vi "Find Connection.vi"(9 "Z":dbl, 10 "X":dbl, 11 "All Lines":T1) -> (0 "Distance to nearest":dbl, 1 "Index on Line":i32, 2 "Nearest Line":i32, 3 "Line found?":bool, 4 "Bool to number":u32, 5 "Z Coonnection":dbl, 7 "X Connection":dbl)   [LabVIEW 2014, in "Map Data.lvlib"]
uses:
  Map Data.lvlib
  All-Lines.ctl
  LineCluster.ctl
  LineConnection.ctl
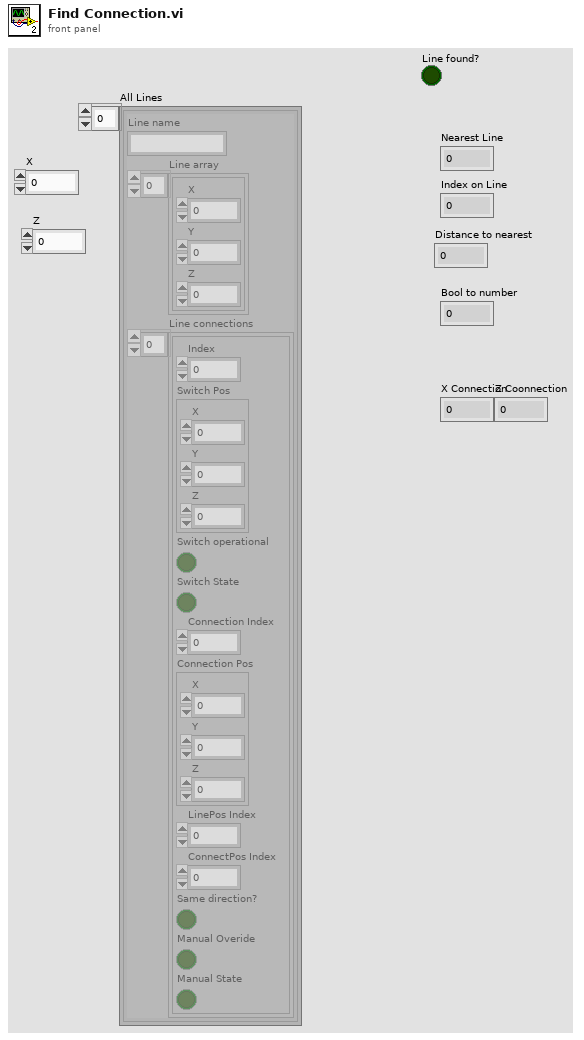
[diagram p1: front panel]
types:
  T1 = typedef "Map Data.lvlib/All-Lines.ctl" = T2[]
  T2 = typedef "Map Data.lvlib/LineCluster.ctl" = cluster{"Line name":string, "Line array":cluster{"X":dbl, "Y":dbl, "Z":dbl}[], "Line connections":T3[]}
  T3 = typedef "Map Data.lvlib/LineConnection.ctl" = cluster{"Index":i32, "Switch Pos":cluster{"X":dbl, "Y":dbl, "Z":dbl}, "Switch operational":bool, "Switch State":bool, "Connection Index":i32, "Connection Pos":cluster{"X":dbl, "Y":dbl, "Z":dbl}, "LinePos Index":i32, "ConnectPos Index":i32, "Same direction?":bool, "Manual Overide":bool, "Manual State":bool}
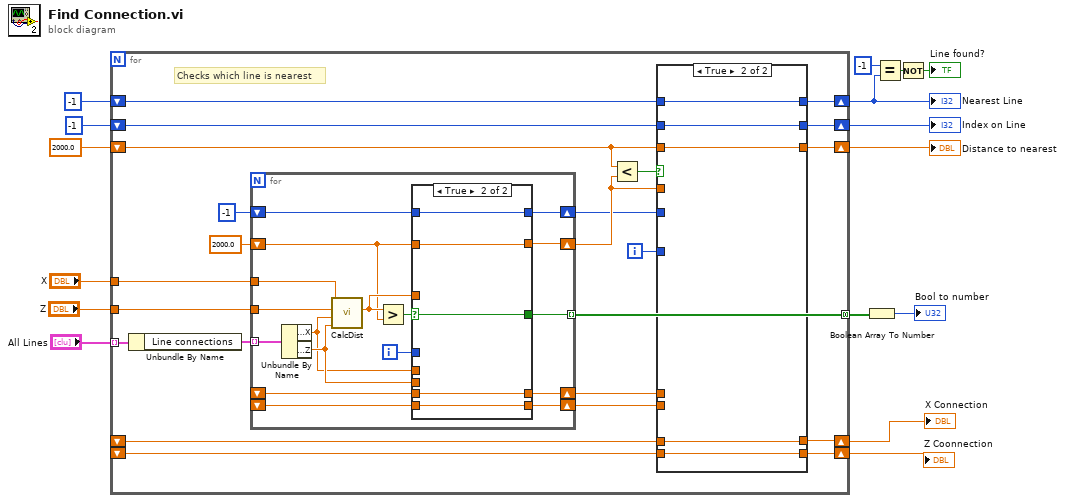
[diagram p0: block diagram]
diagram:
  n1 = for {
    tunnel: "All Lines" -> [w39] mode=indexing
    tunnel: "X" -> [w37]
    tunnel: "Z" -> [w36]
    shift-right: [w34] -> w14
    shift-left: 2000.0 ("Distance") -> [w30]
    shift-right: [w32] -> w10
    shift-left: -1 -> [w31]
    shift-right: [w24] -> w5
    shift-left: -1 -> [w27]
    tunnel: [w23] -> w4 mode=concatenating
    shift-right: [w20] -> w1
    shift-left: _ -> [w17]
    shift-right: [w19] -> w2
    shift-left: _ -> [w18]
    i -> [w33]
    # "Checks which line is nearest"
    n2 = Unbundle By Name(w39) -> ("Line connections"=w38:T3[])
    n3 = for {
      tunnel: w37 -> [w66]
      tunnel: w38 -> [w65] mode=indexing
      tunnel: w36 -> [w63]
      shift-right: [w61] -> w29
      shift-left: 2000.0 ("Distance") -> [w56]
      shift-right: [w58] -> w25
      shift-left: -1 -> [w60]
      tunnel: [w57] -> w23 mode=indexing
      shift-right: [w54] -> w22
      shift-left: _ -> [w50]
      shift-right: [w52] -> w21
      shift-left: _ -> [w51]
      i -> [w59]
      n4 = Unbundle By Name(w65) -> ("Switch Pos.X"=w53:dbl, "Switch Pos.Z"=w55:dbl)
      n5 = call "CalcDist.vi"("Y2"=w55, "X2"=w53, "Y1"=w63, "X1"=w66) -> ("Distance"=w62:dbl)  [unwired: 7 in]
      n6 = Greater?(x=w62, y=w56) -> (0:w64:bool)
      n7 = case shown="True" w64 {
        selector: w64 -> [w69 w74]
        tunnel: w62 -> [w71 _]
        tunnel: [w71 w76] -> w61
        tunnel: w56 -> [_ w76]
        tunnel: w60 -> [_ w75]
        tunnel: w59 -> [w70 _]
        tunnel: [w70 w75] -> w58
        tunnel: [w69 w74] -> w57
        tunnel: w55 -> [w68 _]
        tunnel: [w68 w72] -> w54
        tunnel: w53 -> [w67 _]
        tunnel: [w67 w73] -> w52
        tunnel: w51 -> [_ w73]
        tunnel: w50 -> [_ w72]
        frame False {
        }
        frame True {
        }
      }
    }
    n8 = Less?(x=w30, y=w29) -> (x < y?=w28:bool)
    n9 = case shown="True" w28 {
      tunnel: w29 -> [w44 _]
      tunnel: [w44 w48] -> w34
      tunnel: w30 -> [_ w48]
      tunnel: w33 -> [w43 _]
      tunnel: [w43 w49] -> w32
      tunnel: w31 -> [_ w49]
      tunnel: w27 -> [_ w47]
      tunnel: w25 -> [w42 _]
      tunnel: [w42 w47] -> w24
      tunnel: w22 -> [w41 _]
      tunnel: w21 -> [w40 _]
      tunnel: [w41 w45] -> w20
      tunnel: [w40 w46] -> w19
      tunnel: w18 -> [_ w46]
      tunnel: w17 -> [_ w45]
      frame False {
      }
      frame True {
      }
    }
  }
  "Nearest Line" <- w10
  "Distance to nearest" <- w14
  "Index on Line" <- w5
  "X Connection" <- w2
  "Z Coonnection" <- w1
  n10 = Boolean Array To Number(Boolean array=w4) -> (number=→"Bool to number":u32)
  n11 = Equal?(x=-1, y=w10) -> (x = y?=w8:bool)
  n12 = Not(x=w8) -> (.not. x?=→"Line found?":bool)
